vi "Configure Measurement Type.vi"(8 "error in (no error)":errorcluster, 9 "Measurement Type (0: \"Average\")":i32(ring) items=["\"Average\"", "\"Peak\"", "\"Peak-to-average ratio\"", "\"Minimum\""], 10 "Mode Type (0: Buffer)":i32(ring) items=["Buffer", "List"], 11 "VISA resource name":refnum<visa-resource-name>) -> (0 "error out":errorcluster, 3 "VISA resource name out":refnum<visa-resource-name>)   [LabVIEW 2018, in "Agilent U2000 Series.lvlib"]
doc: "Sets the measurement type of buffered mode or to be performed.\n\nNote: \nThis VI is only applicable for U2040 X-Series."
uses:
  Agilent U2000 Series.lvlib
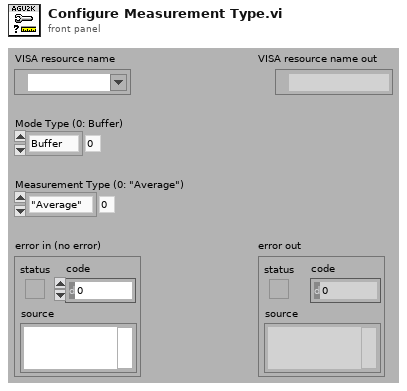
[diagram p1: front panel]
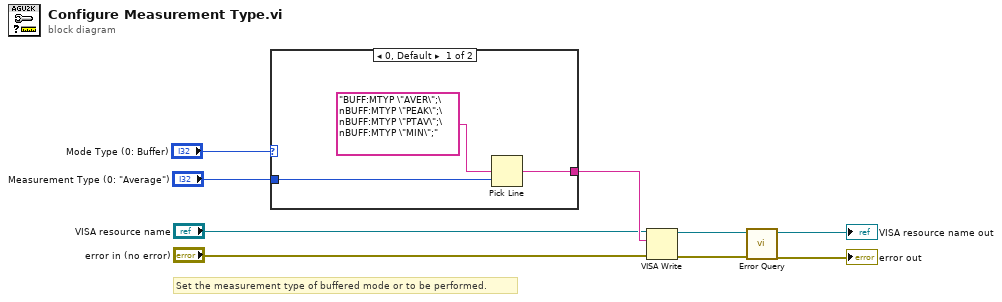
[diagram p0: block diagram]
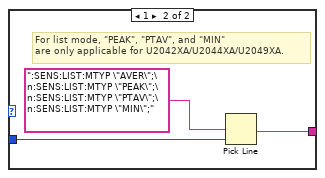
[diagram p2: hidden frame]
diagram:
  # "Set the measurement type of buffered mode or to be performed."
  n1 = case shown="0, Default" "Mode Type (0: Buffer)" {
    tunnel: "Measurement Type (0: \"Average\")" -> [w11 w14]
    tunnel: [w12 w13] -> w4
    frame 0, Default {
      n2 = Pick Line(multi-line string="BUFF:MTYP \"AVER\";\nBUFF:MTYP \"PEAK\";\nBUFF:MTYP \"PTAV\";\nBUFF:MTYP \"MIN\";", line index=w11) -> (output string=w12:string)  [unwired: 1 in]
    }
    frame 1 {
      # "For list mode, \"PEAK\", \"PTAV\", and \"MIN\" \nare only applicable for U2042XA/U2044XA/U2049XA."
      n3 = Pick Line(multi-line string=":SENS:LIST:MTYP \"AVER\";\n:SENS:LIST:MTYP \"PEAK\";\n:SENS:LIST:MTYP \"PTAV\";\n:SENS:LIST:MTYP \"MIN\";", line index=w14) -> (output string=w13:string)  [unwired: 1 in]
    }
  }
  n4 = VISA Write(VISA resource name="VISA resource name", write buffer=w4, error in (no error)="error in (no error)") -> (VISA resource name out=w9:refnum<visa-resource-name>, error out=w8:errorcluster)  [unwired: 1 out]
  n5 = call "Error Query.vi"("error in (no error)"=w8, "VISA resource name"=w9) -> ("error out"=→"error out":errorcluster, "VISA resource name out"=→"VISA resource name out":refnum<visa-resource-name>)  [unwired: 6 in, 2 out]
